vi "Boot Motor Controlers.vi"(8 "error in (no error)":errorcluster, 11 "CANOpen Session in":refnum<k20>) -> (0 "error out":errorcluster, 1 "Left motor Clustered SDO":T1, 2 "Right motor Clustered SDO":T1, 3 "CANOpen Session out":refnum<k20>, 4 "Error":bool)   [LabVIEW 2016]
uses:
  Clustered SDO.ctl
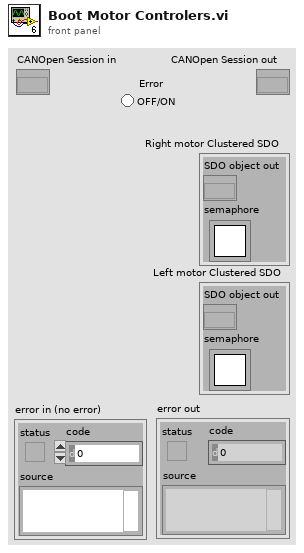
[diagram p1: front panel]
types:
  T1 = typedef "Clustered SDO.ctl" = cluster{"SDO object out":refnum<k20>, "semaphore":T2}
  T2 = typedef "Semaphore RefNum" = refnum<k1>
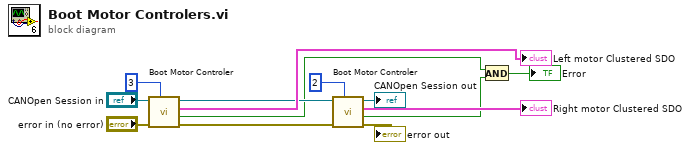
[diagram p0: block diagram]
diagram:
  n1 = call "Boot Motor Controler.vi"("Node ID"=u8 3, "error in (no error)"="error in (no error)", "CANOpen Session in"="CANOpen Session in") -> ("error out"=w8:errorcluster, "Success?"=w7:bool, "Clustered SDO"=→"Left motor Clustered SDO":T1, "CANOpen Session out"=w10:refnum<k20>)  [unwired: 5 in]
  n2 = call "Boot Motor Controler.vi"("Node ID"=u8 2, "error in (no error)"=w8, "CANOpen Session in"=w10) -> ("error out"=→"error out":errorcluster, "Success?"=w6:bool, "Clustered SDO"=→"Right motor Clustered SDO":T1, "CANOpen Session out"=→"CANOpen Session out":refnum<k20>)  [unwired: 5 in]
  n3 = And(x=w7, y=w6) -> (x .and. y?=→"Error":bool)
